vi "Initialize Widget.vi"(8 "widget identification":string, 9 "result":bool, 10 "time / date":timestamp) -> (3 "widget test results out":refnum<class "Widget Test Results.lvclass">)   [LabVIEW 2020, in "Widget Test Results.lvclass"]
doc: "This VI initializes the data members of the class \"Widget Test Results Parent Class.\""
uses:
  Widget Test Results.lvclass
  Widget Test Results.lvclass/Widget Test Results.ctl
  Test Results/Test Results Base Class.lvclass
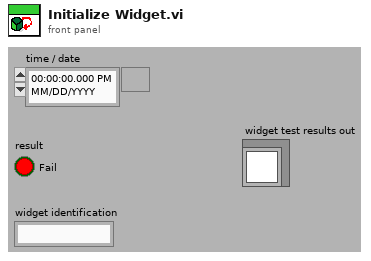
[diagram p1: front panel]
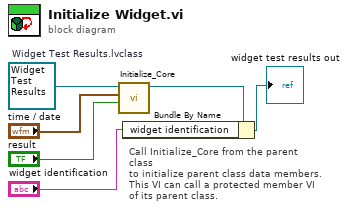
[diagram p0: block diagram]
diagram:
  w2 = refnum<class "Widget Test Results.lvclass"> refnum  # Widget Test Results.lvclass
  # "Call Initialize_Core from the parent class \nto initialize parent class data members. \nThis VI can call a protected member VI \nof its parent class."
  n1 = call "Initialize_Core.vi"("result"="result", "time/date"="time / date", "Test Results \nParent Class in"=w2) -> ("Test Results\nParent Class out"=w1:refnum<class "Widget Test Results.lvclass">)  [unwired: 8 in]
  n2 = Bundle By Name(cluster=w1, "widget identification"="widget identification") -> (→"widget test results out":refnum<class "Widget Test Results.lvclass">)
